vi "Open_6_Rtoom.vi"(7 "error in (no error)":errorcluster, 10 "Motor Settings":T1={"Rear Left Motor"={"Inversion"=TRUE, "PWM Channel"=enum."PWM 0"}, "Middle Left Motor"={"Inversion"=TRUE, "PWM Channel"=enum."PWM 1"}, "Front Left Motor"={"Inversion"=TRUE, "PWM Channel"=enum."PWM 2"}, "Rear Right Motor"={"Inversion"=FALSE, "PWM Channel"=enum."PWM 3"}, "Middle Right Motor"={"Inversion"=FALSE, "PWM Channel"=enum."PWM 4"}, "Front Right Motor"={"Inversion"=FALSE, "PWM Channel"=enum."PWM 5"}}) -> (0 "error out":errorcluster, 3 "RobotDriveDevRef":T3={"DevStatus"={"status"=FALSE, "code"=0, "source"=""}, "Motors[]"=[], "Square Inputs"=FALSE, "Max Output"=1.0})   [LabVIEW 2017]
doc: "Opens a reference to the robot drive for a four-motor robot using Rev Robotics SPARK motor controllers.\n\nThis software is licensed. Open the labview\\readme\\WPI Robotics Library Open Source License.txt file for more information."
uses:
  <vilib>/Rock Robotics/WPI/RobotDrive/WPI_RobotDriveDevRef.ctl
  <vilib>/Rock Robotics/WPI/MotorControl/WPI_MotorControlDeviceRef.ctl
  <vilib>/Rock Robotics/WPI/MotorControl/WPI_MotorControlType.ctl
  <vilib>/Rock Robotics/SystemInterfaces/DIO/FPGA_DIOPWMChannel.ctl
  <vilib>/Rock Robotics/WPI/PWM/WPI_PWMDeadband.ctl
  <vilib>/Rock Robotics/SystemInterfaces/DIO/FPGA_DIOChannel.ctl
  Drive/Implementation/Motor Settings.ctl
  <vilib>/Rock Robotics/WPI/SafetyOutput/WPI_SafetyOutputConfigMenu.ctl
  <vilib>/Rock Robotics/WPI/MotorControl/WPI_MotorControlOpen TalonSRX.vi
  <vilib>/Rock Robotics/WPI/MotorControl/WPI_MotorControlOpen Talon.vi
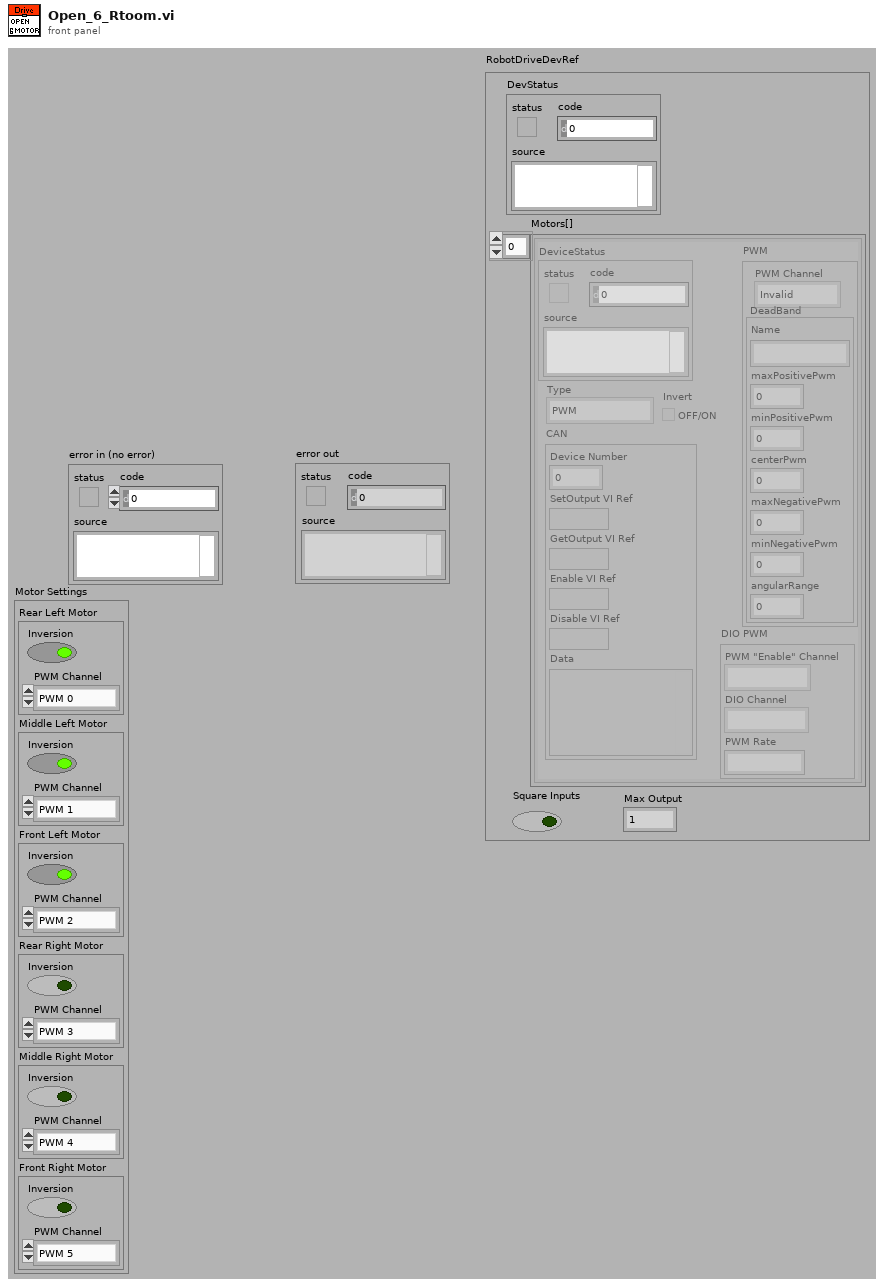
[diagram p1: front panel]
types:
  T1 = typedef "Motor Settings.ctl" = cluster{"Rear Left Motor":cluster{"Inversion":bool, "PWM Channel":T2}, "Middle Left Motor":cluster{"Inversion":bool, "PWM Channel":T2}, "Front Left Motor":cluster{"Inversion":bool, "PWM Channel":T2}, "Rear Right Motor":cluster{"Inversion":bool, "PWM Channel":T2}, "Middle Right Motor":cluster{"Inversion":bool, "PWM Channel":T2}, "Front Right Motor":cluster{"Inversion":bool, "PWM Channel":T2}}
  T2 = typedef "FPGA_DIOPWMChannel.ctl" = enum8{"PWM 0", "PWM 1", "PWM 2", "PWM 3", "PWM 4", "PWM 5", "PWM 6", "PWM 7", "PWM 8", "PWM 9", "PWM MXP 0", "PWM MXP 1", "PWM MXP 2", "PWM MXP 3", "PWM MXP 4", "PWM MXP 5", "PWM MXP 6", "PWM MXP 7", "PWM MXP 8", "PWM MXP 9", "Invalid"}
  T3 = typedef "WPI_RobotDriveDevRef.ctl" = cluster{"DevStatus":errorcluster, "Motors[]":T4[], "Square Inputs":bool, "Max Output":dbl}
  T4 = typedef "WPI_MotorControlDeviceRef.ctl" = cluster{"DeviceStatus":errorcluster, "Type":T5, "PWM":cluster{"PWM Channel":T2, "DeadBand":T6}, "CAN":cluster{"Device Number":u8, "SetOutput VI Ref":variant, "GetOutput VI Ref":variant, "Enable VI Ref":variant, "Disable VI Ref":variant, "Data":variant}, "Invert":bool, "DIO PWM":cluster{"PWM \"Enable\" Channel":T2, "DIOChannel":T7, "PWM Rate":dbl}}
  T5 = typedef "WPI_MotorControlType.ctl" = enum16{"PWM", "CAN", "DIO PWM"}
  T6 = typedef "WPI_PWMDeadband.ctl" = cluster{"Name":string, "maxPositivePwm":i32, "minPositivePwm":i32, "centerPwm":i32, "maxNegativePwm":i32, "minNegativePwm":i32, "angularRange":u16}
  T7 = typedef "FPGA_DIOChannel.ctl" = enum8{"DIO 0", "DIO 1", "DIO 2", "DIO 3", "DIO 4", "DIO 5", "DIO 6", "DIO 7", "DIO 8", "DIO 9", "DIO MXP 0", "DIO MXP 1", "DIO MXP 2", "DIO MXP 3", "DIO MXP 4", "DIO MXP 5", "DIO MXP 6", "DIO MXP 7", "DIO MXP 8", "DIO MXP 9", "DIO MXP 10", "DIO MXP 11", "DIO MXP 12", "DIO MXP 13", "DIO MXP 14", "DIO MXP 15", "SPI Port CS1", "SPI Port CS2", "SPI Port CS3", "SPI Port MISO", "SPI Port MOSI", "Invalid"}
  T8 = typedef "WPI_SafetyOutputConfigMenu.ctl" = enum16{"Enable", "Disable"}
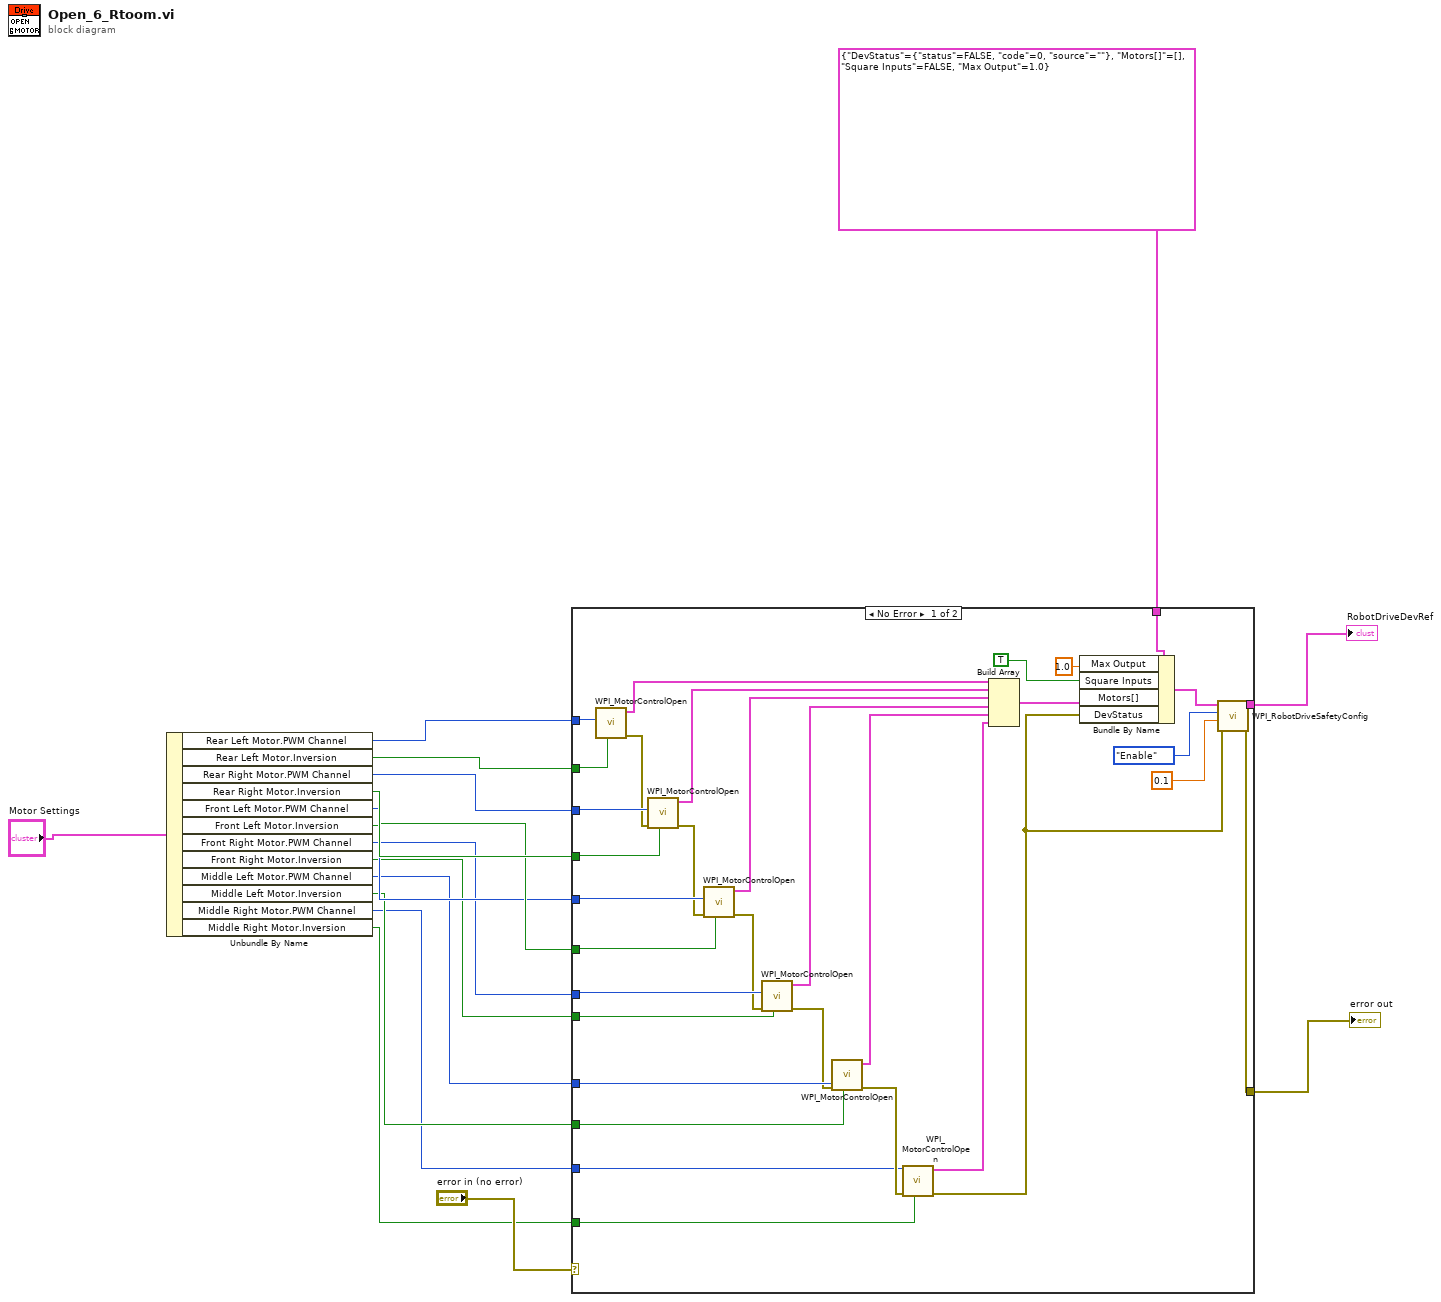
[diagram p0: block diagram]
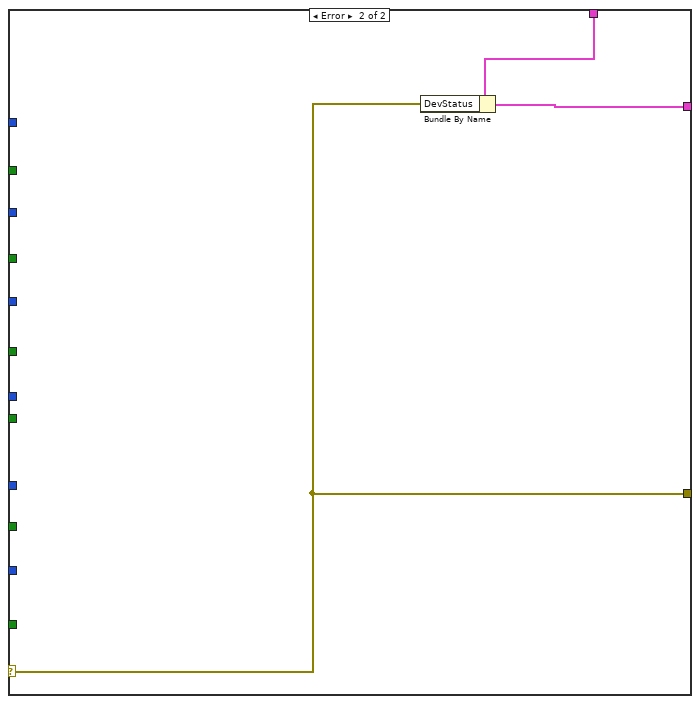
[diagram p2: hidden frame]
diagram:
  n1 = Unbundle By Name("Motor Settings") -> ("Rear Left Motor.PWM Channel"=w11:T2, "Rear Left Motor.Inversion"=w12:bool, "Rear Right Motor.PWM Channel"=w10:T2, "Rear Right Motor.Inversion"=w9:bool, "Front Left Motor.PWM Channel"=w7:T2, "Front Left Motor.Inversion"=w8:bool, "Front Right Motor.PWM Channel"=w6:T2, "Front Right Motor.Inversion"=w1:bool, "Middle Left Motor.PWM Channel"=w5:T2, "Middle Left Motor.Inversion"=w4:bool, "Middle Right Motor.PWM Channel"=w3:T2, "Middle Right Motor.Inversion"=w2:bool)
  n2 = case shown="No Error" "error in (no error)" {
    selector: "error in (no error)" -> [_ w51]
    tunnel: [w30 w52] -> w17
    tunnel: T3 {"DevStatus"={"status"=FALSE, "code"=0, "source"=""}, "Motors[]"=[], "Square Inputs"=FALSE, "Max Output"=1.0} ("RobotDriveDevRef") -> [w50 w53]
    tunnel: w11 -> [w48 _]
    tunnel: w6 -> [w45 _]
    tunnel: w7 -> [w46 _]
    tunnel: w10 -> [w47 _]
    tunnel: w12 -> [w36 _]
    tunnel: w9 -> [w35 _]
    tunnel: w8 -> [w34 _]
    tunnel: [w31 w51] -> w14
    tunnel: w5 -> [w27 _]
    tunnel: w4 -> [w20 _]
    tunnel: w3 -> [w22 _]
    tunnel: w2 -> [w21 _]
    tunnel: w1 -> [w18 _]
    frame No Error {
      n3 = call-poly <vilib>:"WPI_MotorControlOpen.vi"("Invert"=w36, "PWM Channel"=w48) -> ("error out"=w38:errorcluster, "MotorControlDeviceRef"=w44:T4)  [unwired: 2 in, 6 out]
      n4 = call-poly <vilib>:"WPI_MotorControlOpen.vi"("Invert"=w35, "error in (no error)"=w38, "PWM Channel"=w47) -> ("error out"=w39:errorcluster, "MotorControlDeviceRef"=w43:T4)  [unwired: 1 in, 6 out]
      n5 = call-poly <vilib>:"WPI_MotorControlOpen.vi"("Invert"=w34, "error in (no error)"=w39, "PWM Channel"=w46) -> ("error out"=w40:errorcluster, "MotorControlDeviceRef"=w42:T4)  [unwired: 1 in, 6 out]
      n6 = call-poly <vilib>:"WPI_MotorControlOpen.vi"("Invert"=w18, "error in (no error)"=w40, "PWM Channel"=w45) -> ("error out"=w26:errorcluster, "MotorControlDeviceRef"=w41:T4)  [unwired: 1 in, 6 out]
      n7 = call-poly <vilib>:"WPI_MotorControlOpen.vi"("Invert"=w20, "error in (no error)"=w26, "PWM Channel"=w27) -> ("error out"=w24:errorcluster, "MotorControlDeviceRef"=w19:T4)  [unwired: 1 in, 6 out]
      n8 = call-poly <vilib>:"WPI_MotorControlOpen.vi"("Invert"=w21, "error in (no error)"=w24, "PWM Channel"=w22) -> ("error out"=w23:errorcluster, "MotorControlDeviceRef"=w25:T4)  [unwired: 1 in, 6 out]
      n9 = Build Array(w44, w43, w42, w41, w19, w25) -> (w37:T4[])
      n10 = Bundle By Name(cluster=w50, "Max Output"=1.0, "Square Inputs"=TRUE ("DestroyPWM?"), "Motors[]"=w37, "DevStatus"=w23) -> (w32:T3)
      n11 = call <vilib>:"WPI_RobotDriveSafetyConfig.vi"("error in (no error)"=w23, "timeout (s)"=0.1, "mode"=WPI_SafetyOutputConfigMenu."Enable", "RobotDriveDevRef"=w32) -> ("error out"=w31:errorcluster, "RobotDriveDevRef"=w30:T3)  [unwired: 6 out]
    }
    frame Error {
      n12 = Bundle By Name(cluster=w53, "DevStatus"=w51) -> (w52:T3)
    }
  }
  "RobotDriveDevRef" <- w17
  "error out" <- w14
